vi "execute.vi"(8 "error in (no error)":errorcluster, 10 "Context in":refnum<class "Context.lvclass">, 11 "AbortLowerM1M3Command in":refnum<class "AbortLowerM1M3Command.lvclass">) -> (0 "error out":errorcluster, 2 "Context out":refnum<class "Context.lvclass">, 3 "AbortLowerM1M3Command out":refnum<class "AbortLowerM1M3Command.lvclass">)   [LabVIEW 2016, in "AbortLowerM1M3Command.lvclass"]
uses:
  AbortLowerM1M3Command.lvclass
  Context/Context.lvclass
  AbortLowerM1M3Command.lvclass/AbortLowerM1M3Command.ctl
  Context/Context.lvclass/Context.ctl
  Context/getModel.vi
  Context/setModel.vi
  Model/getState.vi
  States/State/State.lvclass
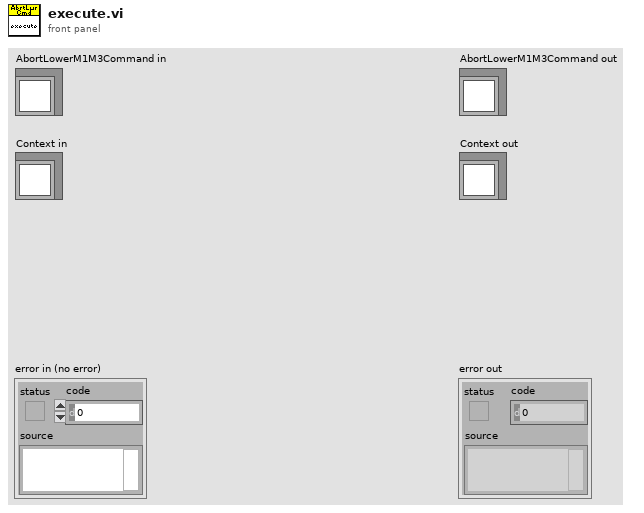
[diagram p1: front panel]
types:
  T1 = typedef "M1M3SupportTopics.lvlib/CommandAbortLowerM1M3.ctl" = cluster{"CommandId":T2, "AbortLowerM1M3":bool}
  T2 = typedef "M1M3SupportTopics.lvlib/CommandId.ctl" = i32
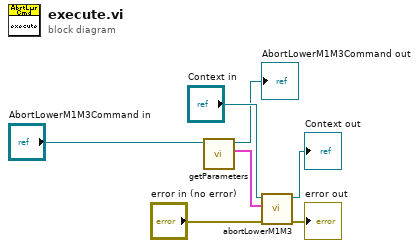
[diagram p0: block diagram]
diagram:
  n1 = call "getParameters.vi"("AbortLowerM1M3Command in"="AbortLowerM1M3Command in") -> ("Parameters"=w6:T1, "AbortLowerM1M3Command out"=→"AbortLowerM1M3Command out":refnum<class "AbortLowerM1M3Command.lvclass">)  [unwired: 9 in]
  n2 = call "abortLowerM1M3.vi"("error in (no error)"="error in (no error)", "Parameters"=w6, "Context in"="Context in") -> ("error out"=→"error out":errorcluster, "Context out"=→"Context out":refnum<class "Context.lvclass">)  [unwired: 7 in]
